vi "Write Current Status Event.vi"(8 "error in":errorcluster, 10 "Current Status":string, 11 "Master Controller in":refnum<class "EMS User Interface.lvclass">) -> (0 "error out":errorcluster, 3 "Master Controller out":refnum<class "EMS User Interface.lvclass">)   [LabVIEW 2018, in "EMS User Interface Actor.lvlib" / "EMS User Interface.lvclass"]
doc: "Sends current status to front panel."
uses:
  EMS User Interface.lvclass
  EMS User Interface.lvclass/EMS User Interface.ctl
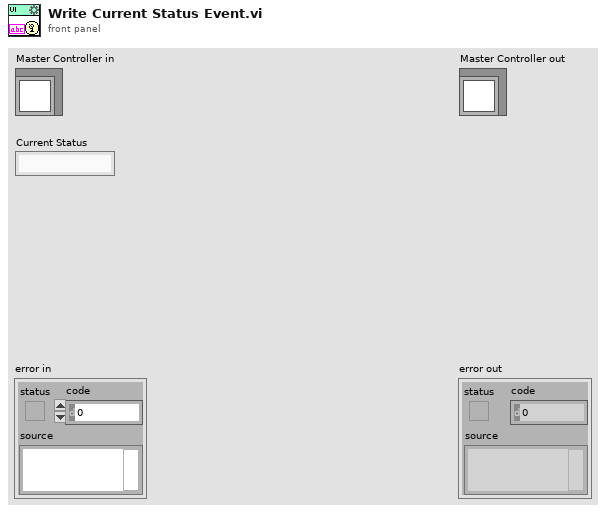
[diagram p1: front panel]
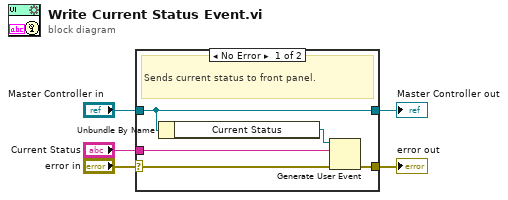
[diagram p0: block diagram]
diagram:
  n1 = case shown="No Error" "error in" {
    selector: "error in" -> [w8 w12]
    tunnel: [w7 w12] -> w4
    tunnel: [w10 w11] -> w2
    tunnel: "Master Controller in" -> [w10 w11]
    tunnel: "Current Status" -> [w6 _]
    frame No Error {
      # "Sends current status to front panel."
      n2 = Unbundle By Name(w10) -> ("Current Status"=w9:refnum<user-event>)
      n3 = Generate User Event(user event=w9, event data cluster=w6, error in=w8) -> (error out=w7:errorcluster)  [unwired: 1 in, 1 out]
    }
    frame Error {
    }
  }
  "error out" <- w4
  "Master Controller out" <- w2
